vi "Configure Reference Oscillator.vi"(6 "External Frequency (10 MHz)":dbl=10000000.0, 7 "Internal BBG Frequency (10 MHz)":dbl=10000000.0, 8 "error in (no error)":errorcluster, 9 "External Bandwidth (25 Hz)":dbl=25.0, 10 "Internal Bandwidth (25 Hz)":dbl=25.0, 11 "VISA resource name":refnum<visa-resource-name>) -> (0 "error out":errorcluster, 3 "VISA resource name out":refnum<visa-resource-name>)   [LabVIEW 2018, in "Agilent PSG MXG Series.lvlib"]
doc: "Configures internal bandwidth, internal BBG frequency, external bandwidth and external frequency of the reference oscillator.\n\n<B>Notes:</B>\n(1) This VI is valid only in E8247C, E8257C, E8267C, E8257D, E8267D, N5161A, N5162A, N5181A, N5182A, N5183A, N5171B, N5172B, N5181B, N5182B, N5173B, N5183B."
uses:
  Agilent PSG MXG Series.lvlib
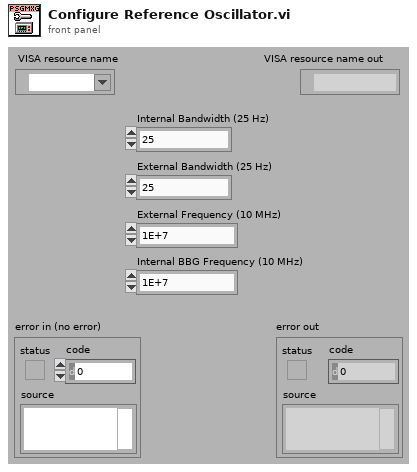
[diagram p1: front panel]
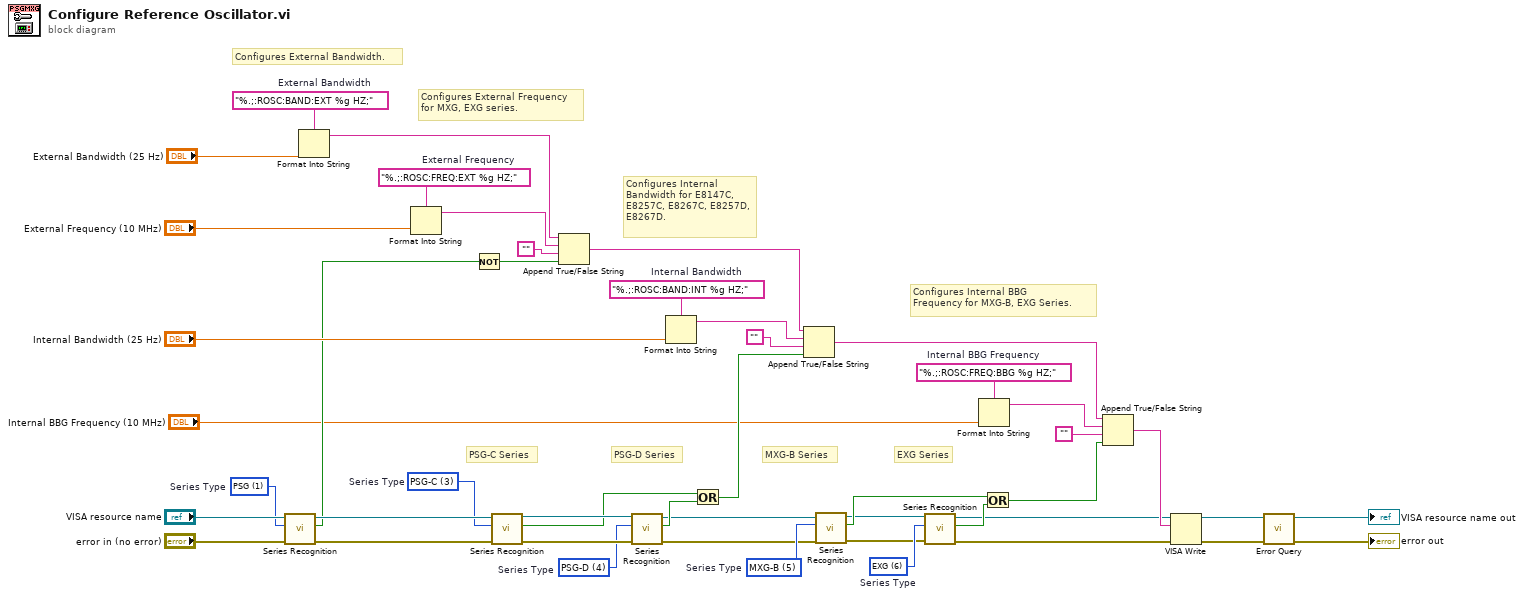
[diagram p0: block diagram]
diagram:
  w14 = u16 6 items=["MXG-A", "PSG", "PSG-A", "PSG-C", "PSG-D", "MXG-B", "EXG"]  # Series Type
  w15 = u16 5 items=["MXG-A", "PSG", "PSG-A", "PSG-C", "PSG-D", "MXG-B", "EXG"]  # Series Type
  w17 = "%.;:ROSC:FREQ:BBG %g HZ;"  # Internal BBG Frequency
  w24 = u16 4 items=["MXG-A", "PSG", "PSG-A", "PSG-C", "PSG-D", "MXG-B", "EXG"]  # Series Type
  w27 = u16 3 items=["MXG-A", "PSG", "PSG-A", "PSG-C", "PSG-D", "MXG-B", "EXG"]  # Series Type
  w33 = u16 1 items=["MXG-A", "PSG", "PSG-A", "PSG-C", "PSG-D", "MXG-B", "EXG"]  # Series Type
  w43 = "%.;:ROSC:FREQ:EXT %g HZ;"  # External Frequency
  w41 = "%.;:ROSC:BAND:INT %g HZ;"  # Internal Bandwidth
  w47 = "%.;:ROSC:BAND:EXT %g HZ;"  # External Bandwidth
  # "EXG Series"
  # "MXG-B Series"
  # "Configures Internal BBG\nFrequency for MXG-B, EXG Series."
  # "PSG-D Series"
  # "PSG-C Series"
  # "Configures Internal\nBandwidth for E8147C,\nE8257C, E8267C, E8257D,\nE8267D."
  # "Configures External Frequency\nfor MXG, EXG series."
  # "Configures External Bandwidth."
  n1 = call "Series Recognition.vi"("error in (no error)"="error in (no error)", "Series Type (0: MXG)"=w33, "VISA resource name"="VISA resource name") -> ("error out"=w34:errorcluster, "Is Series Correct"=w28:bool, "VISA resource name out"=w36:refnum<visa-resource-name>)  [unwired: 1 in, 5 out]
  n2 = Format Into String(format string=w47, "External Bandwidth (25 Hz)") -> (resulting string=w32:string)  [unwired: 2 in, 1 out]
  n3 = Format Into String(format string=w43, "External Frequency (10 MHz)") -> (resulting string=w31:string)  [unwired: 2 in, 1 out]
  n4 = Not(x=w28) -> (.not. x?=w29:bool)
  n5 = call "Series Recognition.vi"("error in (no error)"=w34, "Series Type (0: MXG)"=w27, "VISA resource name"=w36) -> ("error out"=w25:errorcluster, "Is Series Correct"=w20:bool, "VISA resource name out"=w26:refnum<visa-resource-name>)  [unwired: 1 in, 5 out]
  n6 = Append True/False String(1:w29, 2:"", 3:w31, 4:w32) -> (0:w23:string)
  n7 = call "Series Recognition.vi"("error in (no error)"=w25, "Series Type (0: MXG)"=w24, "VISA resource name"=w26) -> ("error out"=w3:errorcluster, "Is Series Correct"=w21:bool, "VISA resource name out"=w6:refnum<visa-resource-name>)  [unwired: 1 in, 5 out]
  n8 = Format Into String(format string=w41, "Internal Bandwidth (25 Hz)") -> (resulting string=w22:string)  [unwired: 2 in, 1 out]
  n9 = Or(x=w20, y=w21) -> (x .or. y?=w19:bool)
  n10 = Append True/False String(1:w19, 2:"", 3:w22, 4:w23) -> (0:w11:string)
  n11 = call "Series Recognition.vi"("error in (no error)"=w3, "Series Type (0: MXG)"=w15, "VISA resource name"=w6) -> ("error out"=w2:errorcluster, "Is Series Correct"=w12:bool, "VISA resource name out"=w5:refnum<visa-resource-name>)  [unwired: 1 in, 5 out]
  n12 = call "Series Recognition.vi"("error in (no error)"=w2, "Series Type (0: MXG)"=w14, "VISA resource name"=w5) -> ("error out"=w1:errorcluster, "Is Series Correct"=w13:bool, "VISA resource name out"=w4:refnum<visa-resource-name>)  [unwired: 1 in, 5 out]
  n13 = Format Into String(format string=w17, "Internal BBG Frequency (10 MHz)") -> (resulting string=w10:string)  [unwired: 2 in, 1 out]
  n14 = Or(x=w12, y=w13) -> (x .or. y?=w8:bool)
  n15 = Append True/False String(1:w8, 2:"", 3:w10, 4:w11) -> (0:w7:string)
  n16 = VISA Write(VISA resource name=w4, write buffer=w7, error in (no error)=w1) -> (VISA resource name out=w46:refnum<visa-resource-name>, error out=w45:errorcluster)  [unwired: 1 out]
  n17 = call "Error Query.vi"("error in (no error)"=w45, "VISA resource name"=w46) -> ("error out"=→"error out":errorcluster, "VISA resource name out"=→"VISA resource name out":refnum<visa-resource-name>)  [unwired: 8 out]
